vi "ProcessUDPValues.vi"(5 "Event Info":T1, 6 "error in (no error)":errorcluster, 9 "connection ID":refnum<k16>) -> ()   [LabVIEW 2017]
uses:
  <vilib>/Utility/file.llb/Write Delimited Spreadsheet (string).vi
panel:
  out "ProcessTime":dbl
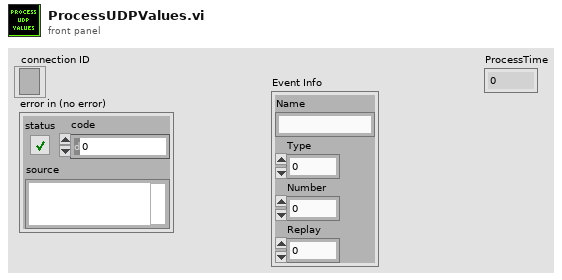
[diagram p1: front panel]
types:
  T1 = cluster{"Name":string, "Type":u8, "Number":u16, "Replay":u8}
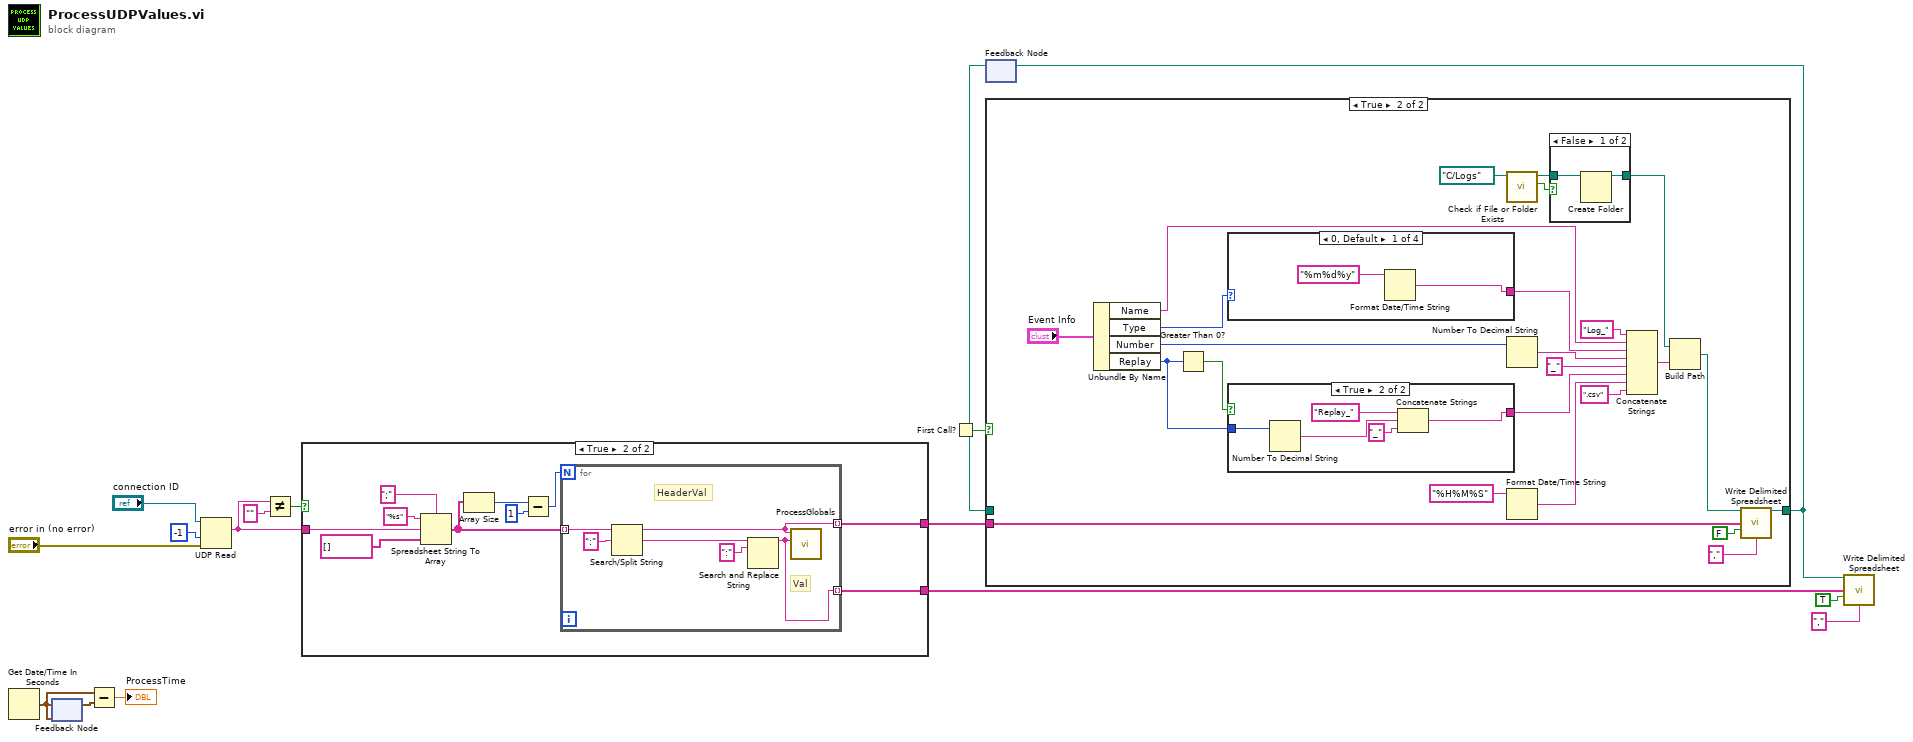
[diagram p0: block diagram]
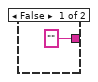
[diagram p4: hidden frame]
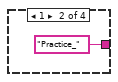
[diagram p5: hidden frame]
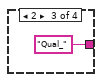
[diagram p6: hidden frame]
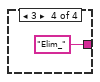
[diagram p7: hidden frame]
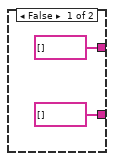
[diagram p8: hidden frame]
diagram:
  n1 = Get Date/Time In Seconds() -> (seconds since 1Jan1904=w14:timestamp)
  n2 = feedback-in #1(w14) -> ()
  n3 = feedback #1(w14) -> (w16:timestamp)
  n4 = Subtract(x=w14, y=w16) -> (x-y=→"ProcessTime":dbl)
  n5 = UDP Read(connection ID="connection ID", timeout ms (25000)=-1, 8:"error in (no error)") -> (data out=w8:string)  [unwired: 1 in, 4 out]
  n6 = Not Equal?(x=w8, y="") -> (x != y?=w9:bool)
  n7 = case shown="True" w9 {
    tunnel: w8 -> [_ w28]
    tunnel: [string[] [] w20] -> w2
    tunnel: [string[] [] w19] -> w1
    frame False {
    }
    frame True {
      n8 = Spreadsheet String To Array(delimiter (Tab)=";" ("search string/char (-)"), format string="%s", spreadsheet string=w28, array type (2D Dbl)=string[] []) -> (array=w24:string[])
      n9 = Array Size(array=w24) -> (size(s)=w23:i32)
      n10 = Subtract(x=w23, y=1) -> (x-y=w21:i32)
      n11 = for {
        N: w21 -> [_]
        tunnel: w24 -> [w34] mode=indexing
        tunnel: [w30] -> w20 mode=indexing
        tunnel: [w29] -> w19 mode=indexing
        # "Val"
        # "HeaderVal"
        n12 = Search/Split String(string=w34, search string/char (-)=":") -> (substring before match=w30:string, match + rest of string=w31:string)  [unwired: 1 in, 1 out]
        n13 = Search and Replace String(input string=w31, search string=":" ("replace string (\"\")")) -> (result string=w29:string)  [unwired: 6 in, 3 out]
        n14 = call "ProcessGlobals.vi"("String"=w30, "String 2"=w29) -> ()  [unwired: 8 in]
      }
    }
  }
  n15 = First Call?() -> (First Call?: T/F=w7:bool)
  n16 = feedback #2() -> (w6:path)  [unwired: 1 in]
  n17 = case shown="True" w7 {
    tunnel: [w35 w57] -> w5
    tunnel: w6 -> [w35 _]
    tunnel: w2 -> [_ w36]
    frame False {
    }
    frame True {
      n18 = Unbundle By Name("Event Info") -> ("Name"=w40:string, "Type"=w38:u8, "Number"=w39:u16, "Replay"=w37:u8)
      n19 = Greater Than 0?(x=w37) -> (x > 0?=w54:bool)
      n20 = case shown="0, Default" w38 {
        tunnel: [w69 "Practice_" "Qual_" "Elim_"] -> w52
        frame 0, Default {
          n21 = Format Date/Time String(time format string (%c)="%m%d%y") -> (date/time string=w69:string)  [unwired: 2 in]
        }
        frame 1 {
        }
        frame 2 {
        }
        frame 3 {
        }
      }
      n22 = case shown="True" w54 {
        tunnel: w37 -> [_ w68]
        tunnel: ["" w64] -> w55
        frame False {
        }
        frame True {
          n23 = Number To Decimal String(number=w68) -> (decimal integer string=w66:string)  [unwired: 1 in]
          n24 = Concatenate Strings("Replay_" ("string"), w66, "_" ("string")) -> (w64:string)
        }
      }
      n25 = call <vilib>:"Check if File or Folder Exists.vi"("path"=path "C:/Logs") -> ("file or folder exists?"=w47:bool, "dup path"=w46:path)  [unwired: 8 in, 1 out]
      n26 = Number To Decimal String(number=w39) -> (decimal integer string=w53:string)  [unwired: 1 in]
      n27 = Format Date/Time String(time format string (%c)="%H%M%S") -> (date/time string=w42:string)  [unwired: 2 in]
      n28 = case shown="False" w47 {
        tunnel: w46 -> [w61 w62]
        tunnel: [w60 w62] -> w45
        frame False {
          n29 = Create Folder(path (use dialog)=w61) -> (created path=w60:path)  [unwired: 2 in, 2 out]
        }
        frame True {
        }
      }
      n30 = Concatenate Strings("Log_" ("string"), w40, w52, w53, "_" ("string"), w55, w42, ".csv" ("string")) -> (w56:string)
      n31 = Build Path(base path=w45, name or relative path=w56) -> (appended path=w49:path)
      n32 = call-poly <vilib>:"Write Delimited Spreadsheet.vi"("file path (dialog if empty)"=w49, "1D data"=w36, "append to file? (new file:F)"=FALSE, "delimiter (\\t)"="," ("delimiter (\\t)")) -> ("new file path (Not A Path if cancelled)"=w57:path)  [unwired: 10 in, 1 out]
    }
  }
  n33 = feedback-in #2(w5) -> ()
  n34 = call-poly <vilib>:"Write Delimited Spreadsheet.vi"("file path (dialog if empty)"=w5, "1D data"=w1, "append to file? (new file:F)"=TRUE, "delimiter (\\t)"="," ("delimiter (\\t)")) -> ()  [unwired: 10 in, 2 out]
